vi "Write UDP Configuration.vi"(8 "error in (no error)":errorcluster, 10 "Hardware Configuration":T1={"Device Port Number"=2001, "Device IP"="192.168.1.1.100", "Timeout"=5000, "Port Number"=1234}, 11 "Plugin_UI in":refnum<class "Plugin_UI.lvclass">) -> (0 "error out":errorcluster, 3 "Plugin_UI out":refnum<class "Plugin_UI.lvclass">)   [LabVIEW 2020, in "Plugin.lvlib" / "Plugin_UI.lvclass"]
doc: "Writes UDP configuration"
uses:
  Plugin_UI.lvclass
  UDP Configuration.ctl
  Plugin_UI.lvclass/Plugin_UI.ctl
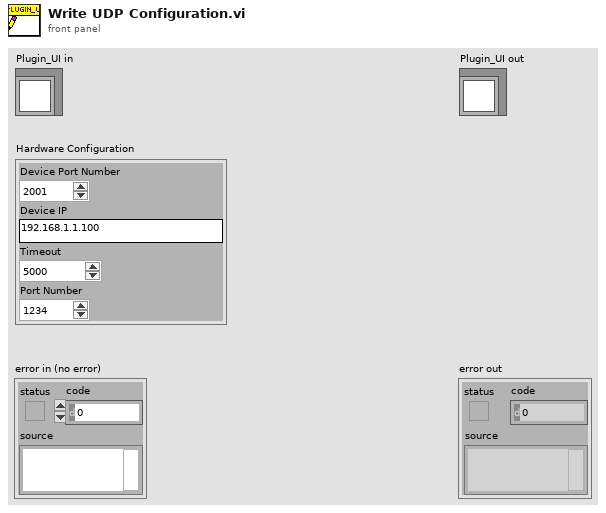
[diagram p1: front panel]
types:
  T1 = typedef "Plugin.lvlib/Plugin_UI.lvclass/UDP Configuration.ctl" = cluster{"Device Port Number":u16, "Device IP":string, "Timeout":i32, "Port Number":u16}
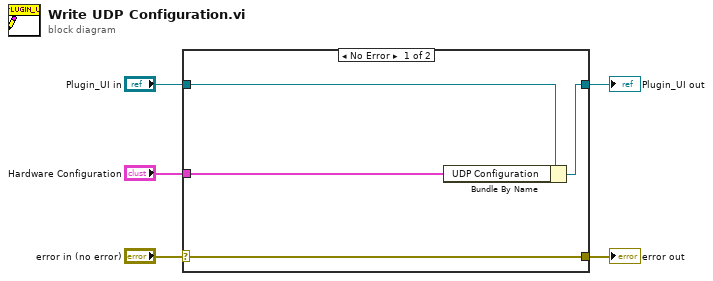
[diagram p0: block diagram]
diagram:
  n1 = case shown="No Error" "error in (no error)" {
    selector: "error in (no error)" -> [w9 w10]
    tunnel: [w9 w10] -> w4
    tunnel: [w7 w11] -> w2
    tunnel: "Plugin_UI in" -> [w8 w11]
    tunnel: "Hardware Configuration" -> [w6 _]
    frame No Error {
      n2 = Bundle By Name(cluster=w8, "UDP Configuration"=w6) -> (w7:refnum<class "Plugin_UI.lvclass">)
    }
    frame Error {
    }
  }
  "error out" <- w4
  "Plugin_UI out" <- w2
